vi "Feed-Position-Graph (SubVI).vi"(10 "Array 2":dbl[](array[numeric]), 11 "Array":dbl[][](array[numeric])) -> (3 "Array 3":cluster{dbl[], dbl[]}[](array[cluster]))   [LabVIEW 2024]
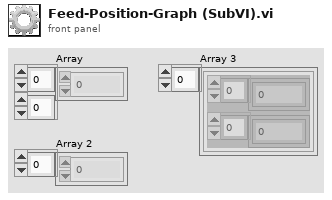
[diagram p1: front panel]
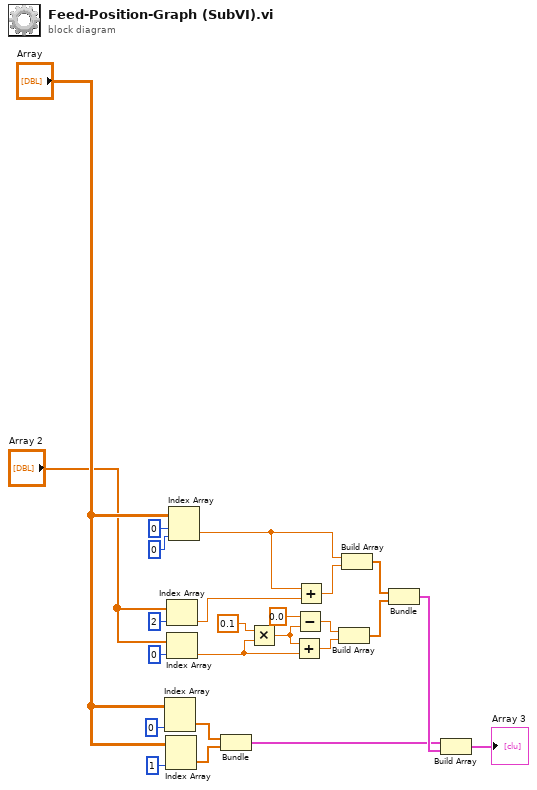
[diagram p0: block diagram]
diagram:
  n1 = Index Array(array="Array", index (col)=0 ("disabled index (col)")) -> (element=w18:dbl[])  [unwired: 1 in]
  n2 = Index Array(array="Array", index (col)=1 ("disabled index (col)")) -> (element=w19:dbl[])  [unwired: 1 in]
  n3 = Index Array(array="Array 2", index=2) -> (element=w7:dbl)
  n4 = Index Array(array="Array 2", index=0) -> (element=w11:dbl)
  n5 = Index Array(array="Array", index (row)=0, index (col)=0) -> (element=w5:dbl)
  n6 = Bundle("Array"=w18, "Array"=w19) -> (w21:cluster{"Array":dbl[], "Array":dbl[]})  [unwired: 1 in]
  n7 = Multiply(x=0.1 ("y"), y=w11) -> (x*y=w13:dbl)
  n8 = Add(x=w13, y=w11) -> (x+y=w15:dbl)
  n9 = Subtract(x=0.0, y=w13) -> (x-y=w14:dbl)
  n10 = Add(x=w5, y=w7) -> (x+y=w4:dbl)
  n11 = Build Array(w14, w15) -> (w6:dbl[])
  n12 = Build Array(w5, w4) -> (w20:dbl[])
  n13 = Bundle(w20, w6) -> (w22:cluster{dbl[], dbl[]})  [unwired: 1 in]
  n14 = Build Array(w21, w22) -> (→"Array 3":cluster{"Array":dbl[], "Array":dbl[]}[])
